vi "Launch graph.vi"(8 "error in (no error)":errorcluster, 9 "Name":string, 10 "MagLabGraph.lvclass":refnum<class "MagLabGraph.lvclass">, 11 "Mag Lab Measure Base in":refnum<class "Mag Lab Measure Base.lvclass">) -> (0 "error out":errorcluster, 2 "Nested Actor's Enqueuer":refnum<class "Message Enqueuer.lvclass">, 3 "Mag Lab Measure Base out":refnum<class "Mag Lab Measure Base.lvclass">)   [LabVIEW 2015, in "Mag Lab Measure Base.lvclass"]
uses:
  Mag Lab Measure Base.lvclass
  Mag Lab Graph/MagLabGraph.lvclass
  <vilib>/ActorFramework/Message Enqueuer/Message Enqueuer.lvclass
  Mag Lab Measure Base.lvclass/Mag Lab Measure Base.ctl
  <vilib>/ActorFramework/Actor/Actor.lvclass
  Mag Lab Error Handler/Mag Lab Error Handler.lvclass
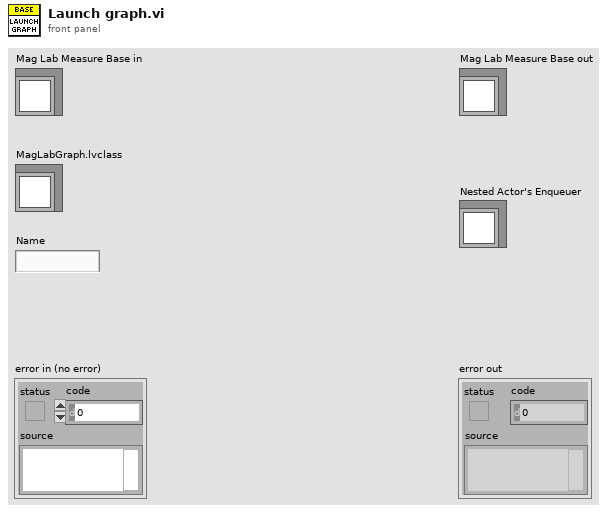
[diagram p1: front panel]
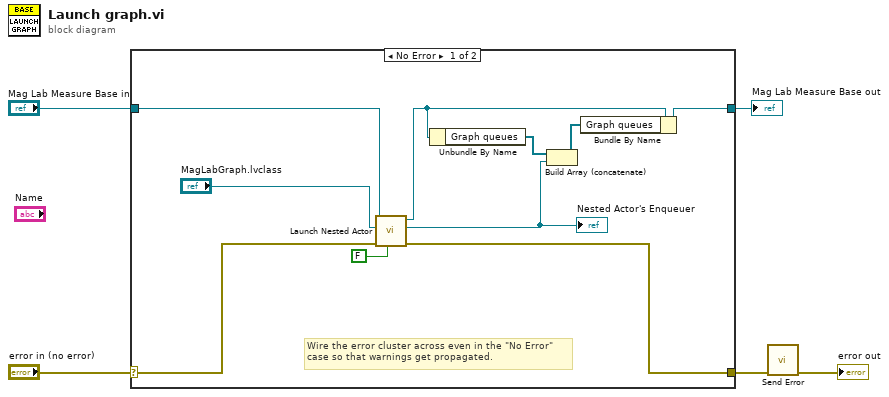
[diagram p0: block diagram]
diagram:
  n1 = case shown="No Error" "error in (no error)" {
    selector: "error in (no error)" -> [w8 w17]
    tunnel: [w6 w17] -> w2
    tunnel: [w10 w16] -> w3
    tunnel: "Mag Lab Measure Base in" -> [w14 w16]
    frame No Error {
      # "Wire the error cluster across even in the \"No Error\"\ncase so that warnings get propagated."
      n2 = call <vilib>:"Launch Nested Actor.vi"("Open Actor Core front panel? (F)"=FALSE, "error in (no error)"=w8, "Nested Actor"="MagLabGraph.lvclass", "Caller Actor in"=w14) -> ("error out"=w6:errorcluster, "Nested Actor's Enqueuer"=w11:refnum<class "Message Enqueuer.lvclass">, "Caller Actor out"=w13:refnum<class "Mag Lab Measure Base.lvclass">)  [unwired: 5 in]
      "Nested Actor's Enqueuer" <- w11
      n3 = Unbundle By Name(w13) -> ("Graph queues"=w12:refnum<class "Message Enqueuer.lvclass">[])
      n4 = Build Array (concatenate)(w12, w11) -> (w9:refnum<class "Message Enqueuer.lvclass">[])
      n5 = Bundle By Name(cluster=w13, "Graph queues"=w9) -> (w10:refnum<class "Mag Lab Measure Base.lvclass">)
    }
    frame Error {
    }
  }
  "Mag Lab Measure Base out" <- w3
  n6 = call "Send Error.vi"("error in (no error)"=w2) -> ("error out"=→"error out":errorcluster)  [unwired: 9 in, 1 out]
